vi "read_pressures.vi"(8 "data task error in":errorcluster, 10 "press task in":refnum<k21>, 11 "Channel 1":tag) -> (0 "press error out":errorcluster, 2 "press task out":refnum<k21>, 3 "Ch. 1 value":dbl format="%0.2f")   [LabVIEW 2014]
uses:
  <vilib>/DAQmx/create/channels.llb/DAQmx Create Channel (AI-Voltage-Basic).vi
  <vilib>/DAQmx/configure/trigger.llb/DAQmx Start Trigger (None).vi
  <vilib>/DAQmx/read.llb/DAQmx Read (Analog 1D DBL NChan 1Samp).vi
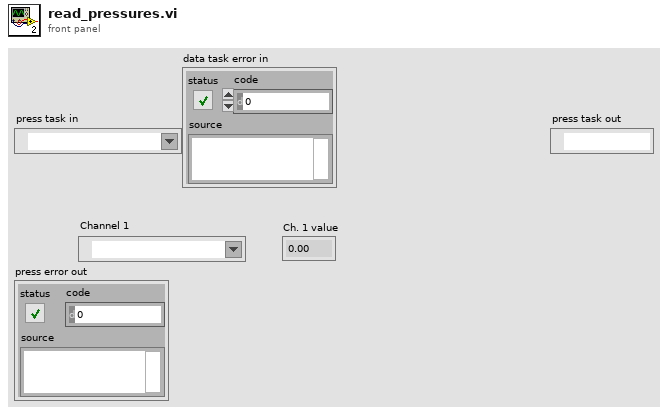
[diagram p1: front panel]
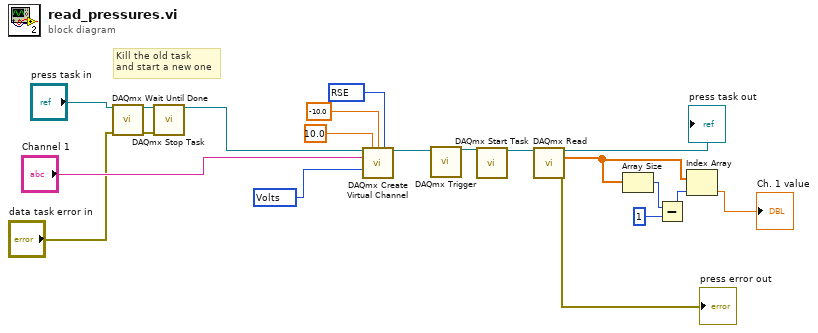
[diagram p0: block diagram]
diagram:
  w15 = 10083 items=["default"=-1, "RSE"=10083, "NRSE"=10078, "Differential"=10106, "Pseudodifferential"=12529] ("input terminal configuration")
  w17 = 10348 items=["Volts"=10348, "From Custom Scale"=10065] ("units")
  # "Kill the old task\nand start a new one"
  n1 = call <vilib>:"DAQmx Wait Until Done.vi"("task/channels in"="press task in", "error in"="data task error in") -> ("task out"=w2:refnum<k21>, "error out"=w1:errorcluster)  [unwired: 12 in]
  n2 = call <vilib>:"DAQmx Stop Task.vi"("task/channels in"=w2, "error in"=w1) -> ("task out"=w12:refnum<k21>)  [unwired: 12 in, 1 out]
  n3 = call-poly <vilib>:"DAQmx Create Virtual Channel.vi"("task in"=w12, "maximum value"=10.0, "minimum value"=-10.0, "input terminal configuration"=w15, "physical channels"="Channel 1", "units"=w17) -> ("task out"=w11:refnum<k21>)  [unwired: 8 in, 1 out]
  n4 = call-poly <vilib>:"DAQmx Trigger.vi"("task/channels in"=w11) -> ("task out"=w10:refnum<k21>)  [unwired: 13 in, 1 out]
  n5 = call <vilib>:"DAQmx Start Task.vi"("task/channels in"=w10) -> ("task out"=w16:refnum<k21>)  [unwired: 13 in, 1 out]
  n6 = call-poly <vilib>:"DAQmx Read.vi"("task/channels in"=w16) -> ("task out"=→"press task out":refnum<k21>, "data"=w9:dbl[], "error out"=→"press error out":errorcluster)  [unwired: 12 in]
  n7 = Array Size(array=w9) -> (size(s)=w8:i32)
  n8 = Subtract(x=w8, y=1) -> (x-y=w6:i32)
  n9 = Index Array(array=w9, index=w6) -> (element=→"Ch. 1 value":dbl)
